vi "Get_ADAM_Ch_names_client.vi"(1 "Channel names set":T1) -> (0 "Ch names":string[](array[string]))   [LabVIEW 2017]
doc: "This is an example of using features of the VI Server as a client. It shows how you might browse from one or more applications that may be exporting data from one or more data stations. \n\nThe example shows how to query a server for its list of exported VIs, how to get references to the VIs, and how call them with the Call By Reference function."
uses:
  Sub VIs/ADAM Controls/Channel_names.ctl
  Anemometry/Anemometry Sub Vis/Controls/Global_mode.ctl
  Sub VIs/ADAM Controls/Channel_State.ctl
  Anemometry/Anemometry Sub Vis/Globals/Preference_global.vi
panel:
  in  "Server type":refnum<vi>
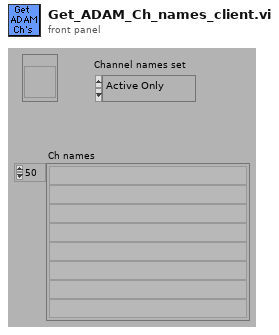
[diagram p1: front panel]
types:
  T1 = typedef "Channel_names.ctl" = enum16{"Active Only", "Active + Off", "All Channels"}
  T2 = typedef "Server_Comms.ctl" = enum16{"Server Link Healthy", "Do Not Link To Server"}
  T3 = typedef "Global_mode.ctl" = enum16{"Read Global", "Load Global From File", "Write Global to File"}
  T4 = typedef "Channel_State.ctl" = enum16{"On", "Off", "Always On", "Always Off"}
  T5 = typedef "Ch_description_ADAM.ctl" = cluster{"Ch Name":string, "Type":T6, "Function":T7, "Ch State":T4, "Calibration type":T8, "A":dbl, "B":dbl, "C":dbl, "D":dbl, "Comments":string, "Address":T9, "String":string, "Duty":u16}
  T6 = typedef "Module_type_ADAM.ctl" = string
  T7 = typedef "Function_ADAM.ctl" = enum16{"Analogue Input", "Digital Input", "Event counter", "Event rate", "Analogue Output", "Digital Output", "Relay Output"}
  T8 = typedef "Calib_type_ADAM.ctl" = string
  T9 = typedef "Address.ctl" = cluster{"Main":i32, "Ch.":i32, "Sub":i32, "Port Name":string}
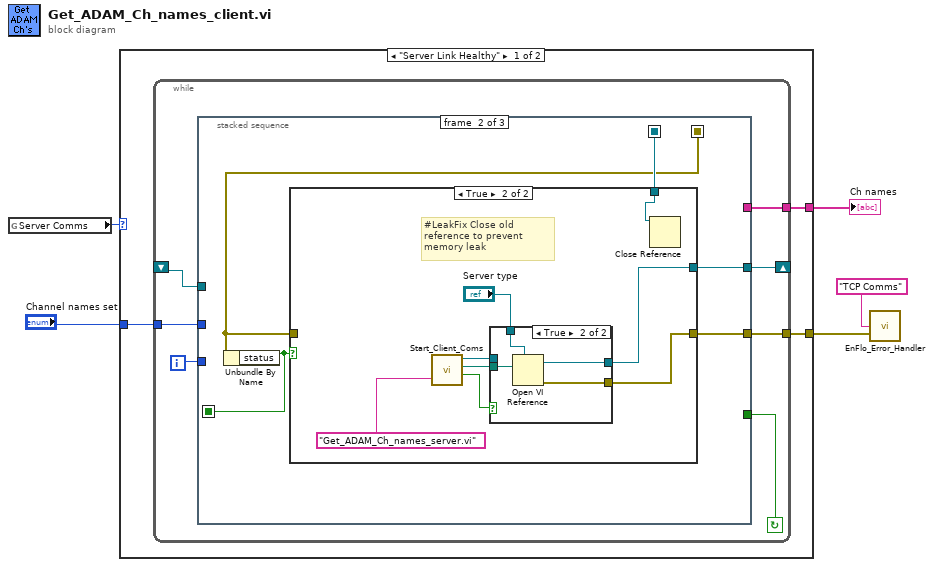
[diagram p0: block diagram]
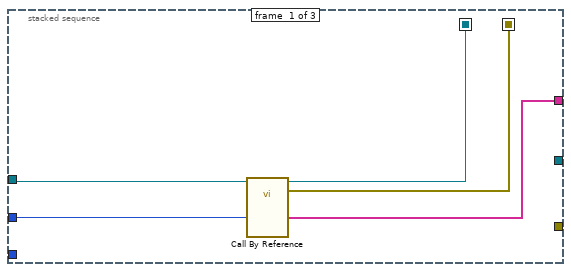
[diagram p2: hidden frame]
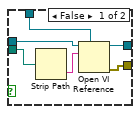
[diagram p4: hidden frame]
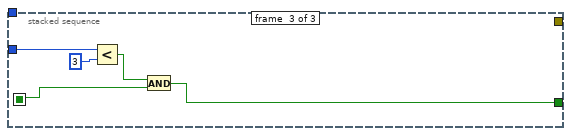
[diagram p5: hidden frame]
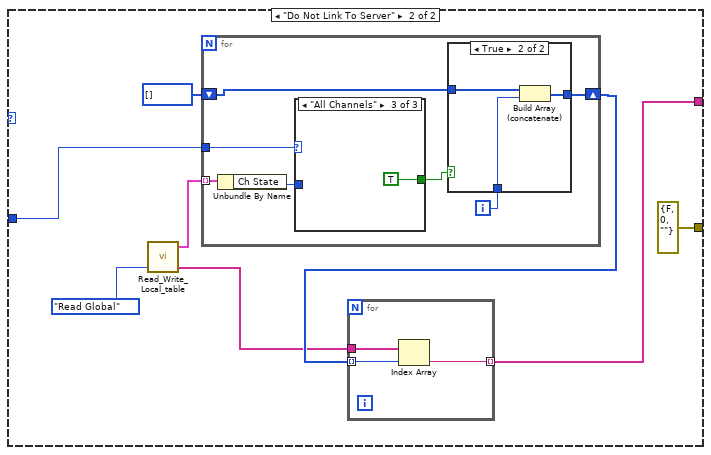
[diagram p6: hidden frame]
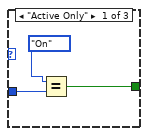
[diagram p8: hidden frame]
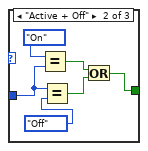
[diagram p9: hidden frame]
diagram:
  n1 = global read "Preference_global.vi" "Server Comms"() -> (w4:T2)
  n2 = case shown="\"Server Link Healthy\"" w4 {
    tunnel: [w8 w51] -> w5
    tunnel: [w7 errorcluster {"status"=FALSE, "code"=0, "source"=""} ("Error IO")] -> w3
    tunnel: "Channel names set" -> [w6 w55]
    frame "Server Link Healthy" {
      n3 = while {
        tunnel: [w10] -> w7
        tunnel: [w11] -> w8
        shift-left: _ -> [w15]
        shift-right: [w14] -> _
        tunnel: w6 -> [w9]
        i -> [w13]
        stop <- w12 continue-if-true
        n4 = stacked-sequence {
          seq-local: [w18 _ _] -> [_ w24 _]
          seq-local: [w17 _ _] -> [_ w21 _]
          seq-local: [_ w23 _] -> [_ _ w47]
          tunnel: w15 -> [w20 _ _]
          tunnel: [_ w25 _] -> w14
          tunnel: w13 -> [_ _ w48]
          tunnel: [_ _ w46] -> w12
          tunnel: [w19 _ _] -> w11
          tunnel: [_ w22 _] -> w10
          tunnel: w9 -> [w16 _ _]
          frame #0 {
            n5 = call-by-ref "?"(reference=w20, "Channel names set"=w16) -> (reference out=w18:refnum<vi>, error out=w17:errorcluster, "Ch names"=w19:string[])  [unwired: 1 in]
          }
          frame #1 {
            n6 = Unbundle By Name(w21) -> ("status"=w23:bool)
            n7 = case shown="True" w23 {
              tunnel: [w27 w31] -> w25
              tunnel: w24 -> [w27 w28]
              tunnel: [w26 w29] -> w22
              tunnel: w21 -> [w26 _]
              frame False {
              }
              frame True {
                # "#LeakFix Close old reference to prevent memory leak"
                n8 = call "Start_Client_Coms.vi"("VI name to run on server"="Get_ADAM_Ch_names_server.vi") -> ("LabVIEW application reference"=w33:refnum<vi>, "Checked VI name"=w34:path, "Local Call"=w32:bool)  [unwired: 1 in, 1 out]
                n9 = case shown="True" w32 {
                  tunnel: [w38 w45] -> w31
                  tunnel: "Server type" -> [w37 w44]
                  tunnel: w34 -> [w41 w43]
                  tunnel: w33 -> [w36 _]
                  tunnel: [w39 w42] -> w29
                  frame False {
                    n10 = Strip Path(path=w41) -> (name=w40:string)  [unwired: 1 out]
                    n11 = Open VI Reference(type specifier VI Refnum (for type only)=w37, application reference (local)=w36, vi path=w40) -> (vi reference=w38:refnum<vi>, error out=w39:errorcluster)  [unwired: 1 in, 2 out]
                  }
                  frame True {
                    n12 = Open VI Reference(type specifier VI Refnum (for type only)=w44, vi path=w43) -> (vi reference=w45:refnum<vi>, error out=w42:errorcluster)  [unwired: 1 in, 3 out]
                  }
                }
                n13 = Close Reference(reference=w28) -> ()  [unwired: 1 in, 1 out]
              }
            }
          }
          frame #2 {
            n14 = Less?(x=w48, y=3) -> (x < y?=w50:bool)
            n15 = And(x=w50, y=w47) -> (x .and. y?=w46:bool)
          }
        }
      }
    }
    frame "Do Not Link To Server" {
      n16 = call "Read_Write_Local_table.vi"("Mode"=Global_mode."Read Global") -> ("Ch Names"=w52:string[], "Channels Descriptions Out"=w56:T5[])  [unwired: 2 in, 1 out]
      n17 = for {
        tunnel: w56 -> [w68] mode=indexing
        tunnel: w55 -> [w67]
        shift-right: [w63] -> w53
        shift-left: i32[] [] -> [w62]
        i -> [w64]
        n18 = Unbundle By Name(w68) -> ("Ch State"=w66:T4)
        n19 = case shown="\"All Channels\"" w67 {
          tunnel: w66 -> [w75 w80 _]
          tunnel: [w73 w76 TRUE] -> w65
          frame "Active Only" {
            n20 = Equal?(x=Channel_State."On" ("Ch State"), y=w75) -> (x = y?=w73:bool)
          }
          frame "Active + Off" {
            n21 = Equal?(x=Channel_State."On" ("Ch State"), y=w80) -> (x = y?=w77:bool)
            n22 = Equal?(x=w80, y=Channel_State."Off" ("Ch State")) -> (x = y?=w78:bool)
            n23 = Or(x=w77, y=w78) -> (x .or. y?=w76:bool)
          }
          frame "All Channels" {
          }
        }
        n24 = case shown="True" w65 {
          tunnel: w64 -> [_ w72]
          tunnel: [w69 w71] -> w63
          tunnel: w62 -> [w69 w70]
          frame False {
          }
          frame True {
            n25 = Build Array (concatenate)(w70, w72) -> (w71:i32[])
          }
        }
      }
      n26 = for {
        tunnel: w53 -> [w61] mode=indexing
        tunnel: w52 -> [w60]
        tunnel: [w59] -> w51 mode=indexing
        n27 = Index Array(array=w60, index=w61) -> (element=w59:string)
      }
    }
  }
  "Ch names" <- w5
  n28 = call "EnFlo_Error_Handler.vi"("error in (no error)"=w3, "Error Type"="TCP Comms") -> ()  [unwired: 1 in, 3 out]
